vi "Network_Main.vi"(8 "error in (no error)":errorcluster, 11 "DevInfo":T1={"Hostname"="", "IPAddress"="", "MAC"="", "SerialNum"="", "Model"="", "Status"="", "FW"="", "OSDesc"="", "ImgTitle"="", "ImgDesc"="", "ImgVer"="", "ImgID"="", "IP Address Request Mode"=1, "SubnetMask"="", "Gateway"="", "DNSServer"=""} {"IP Address Request Mode" items=["Static"=1, "DHCP/Link-Local"=2, "Link-Local Only"=4, "DHCP Only"=8]}) -> (0 "error out":errorcluster, 3 "Cancelled":bool)   [LabVIEW 2021]
uses:
  TypeDefs/DevInfo.ctl
  1feb173d-b457-4ebd-b016-741c425a2058.vi
  3503507e-3d8e-4ae6-b018-2cfbcbcbc3e1.vi
  7f23f98b-f62e-4c84-a499-f9e01871bdb8.vi
  d7740b82-8dfd-4b86-b168-3c102f68faa4.vi
  36928e67-3434-4745-8582-0b47ffec617e.vi
  333e741c-c09c-4afd-acb8-9a738d66323c.vi
  7c5289c9-eb46-4be9-a5cb-af584f789a3a.vi
  ee792d3c-066e-446b-8644-9ff67b395601.vi
  <userlib>/S2 Labs/Error Reporting/ER Global.vi
  <userlib>/S2 Labs/Error Reporting/Error Reporting Class/subVIs/Report Error.vi
panel:
  in  "Cancel":bool
  in  "Apply Settings":bool
  in  "IP Mode":i32(ring) items=["Static"=1, "DHCP/Link-Local"=2, "Link-Local Only"=4, "DHCP Only"=8]
  in  "DNS.4":u8
  in  "DNS.3":u8
  in  "DNS.2":u8
  in  "DNS.1":u8 caption="DNS"
  in  "GW.4":u8
  in  "GW.3":u8
  in  "GW.2":u8
  in  "GW.1":u8 caption="Gateway"
  in  "Mask.4":u8
  in  "Mask.3":u8
  in  "Mask.2":u8
  in  "Mask.1":u8 caption="Subnet Mask"
  in  "IP.4":u8
  in  "IP.3":u8
  in  "IP.2":u8
  in  "IP.1":u8 caption="IP Address"
  in  "Hostname":string
  # "."
  # "."
  # "."
  # "."
  # "."
  # "."
  # "."
  # "."
  # "."
  # "."
  # "."
  # "."
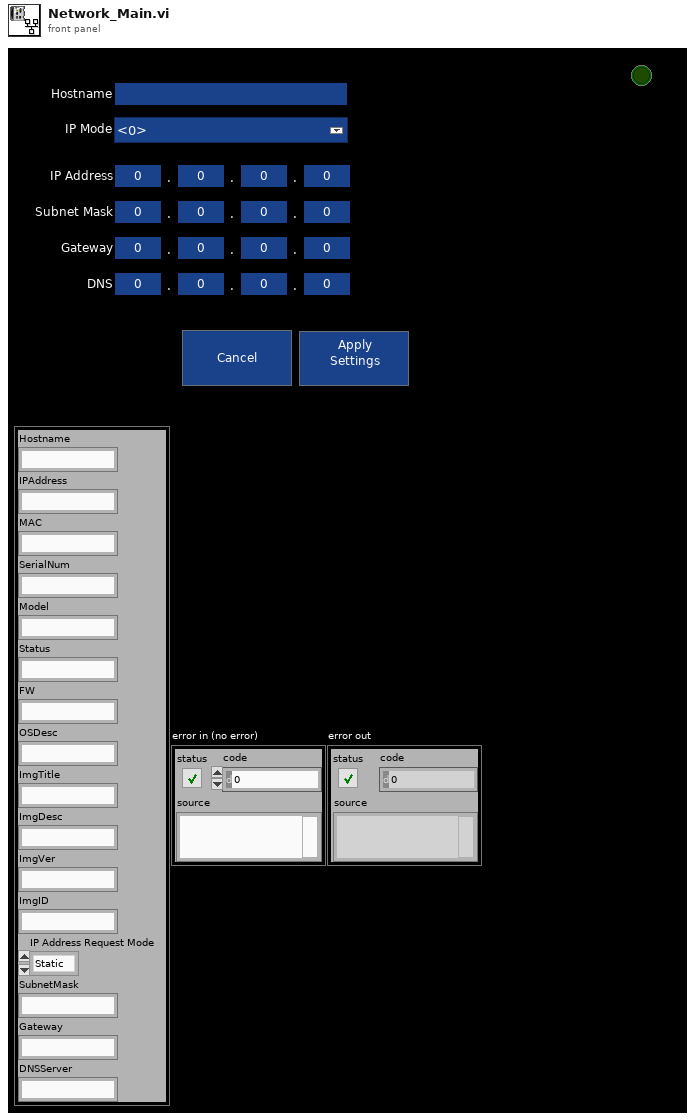
[diagram p1: front panel]
types:
  T1 = typedef "DevInfo.ctl" = cluster{"Hostname":string, "IPAddress":string, "MAC":string, "SerialNum":string, "Model":string, "Status":string, "FW":string, "OSDesc":string, "ImgTitle":string, "ImgDesc":string, "ImgVer":string, "ImgID":string, "IP Address Request Mode":i32, "SubnetMask":string, "Gateway":string, "DNSServer":string}
  T2 = enum8{"Enabled", "Disabled", "Disabled and Grayed Out"}
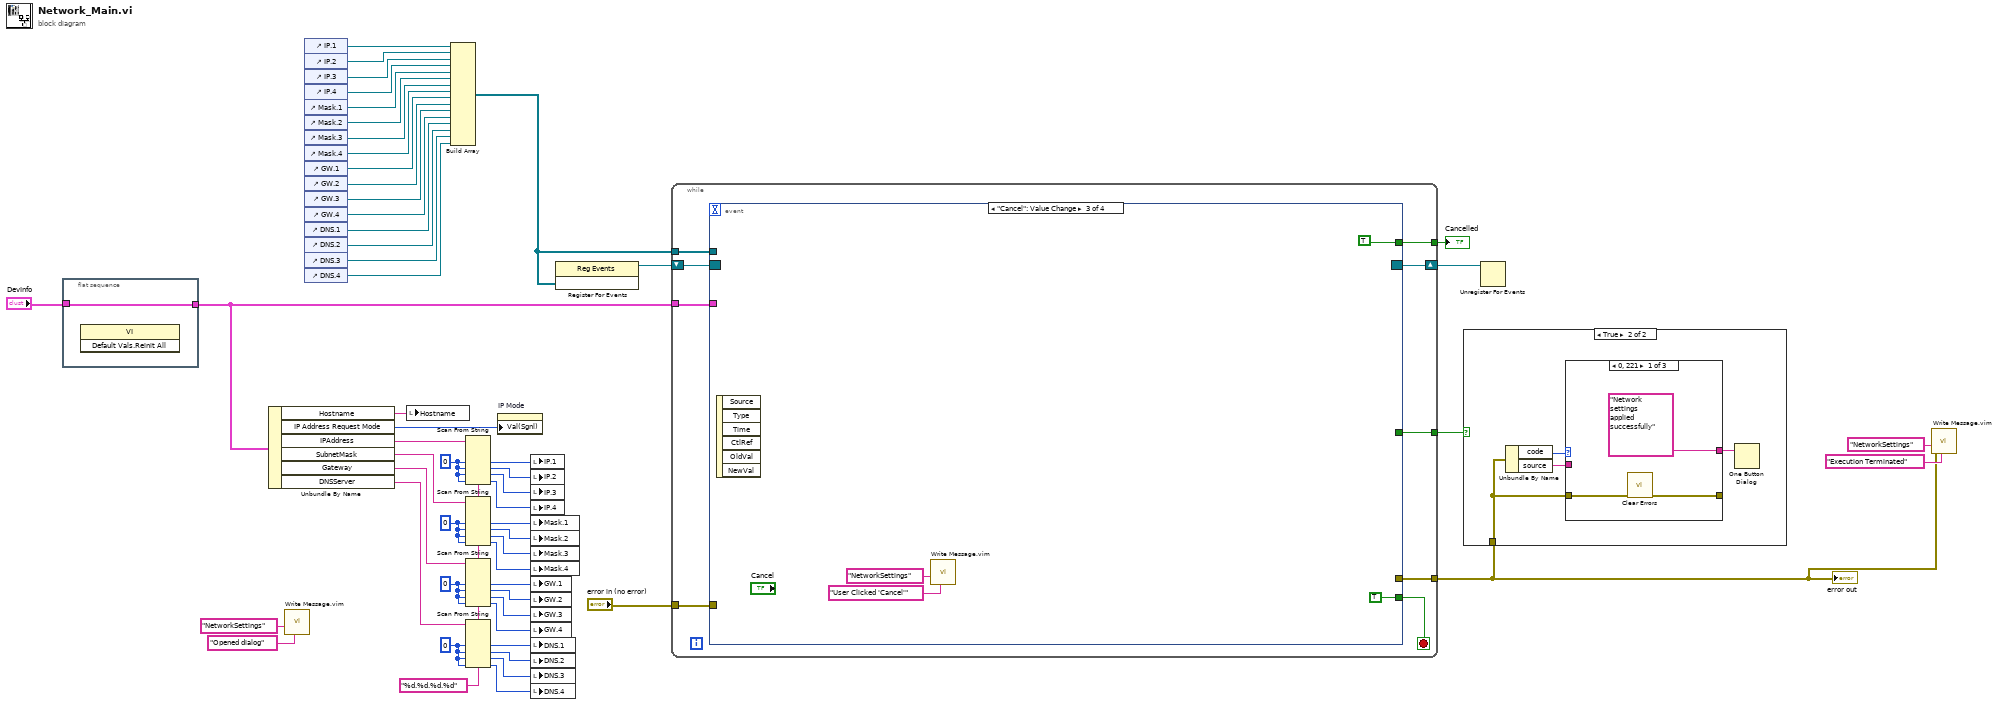
[diagram p0: block diagram]
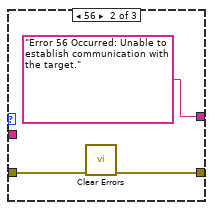
[diagram p3: hidden frame]
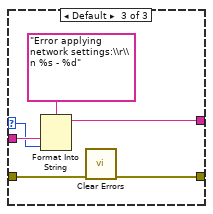
[diagram p4: hidden frame]
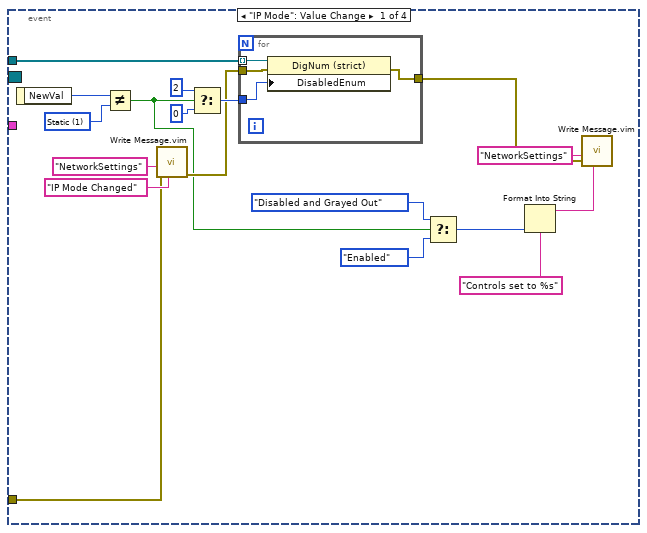
[diagram p5: hidden frame]
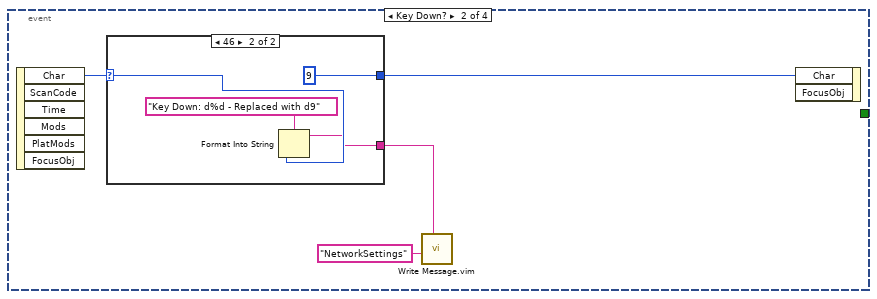
[diagram p6: hidden frame]
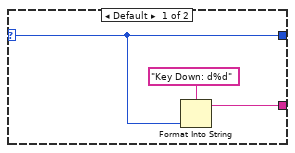
[diagram p7: hidden frame]
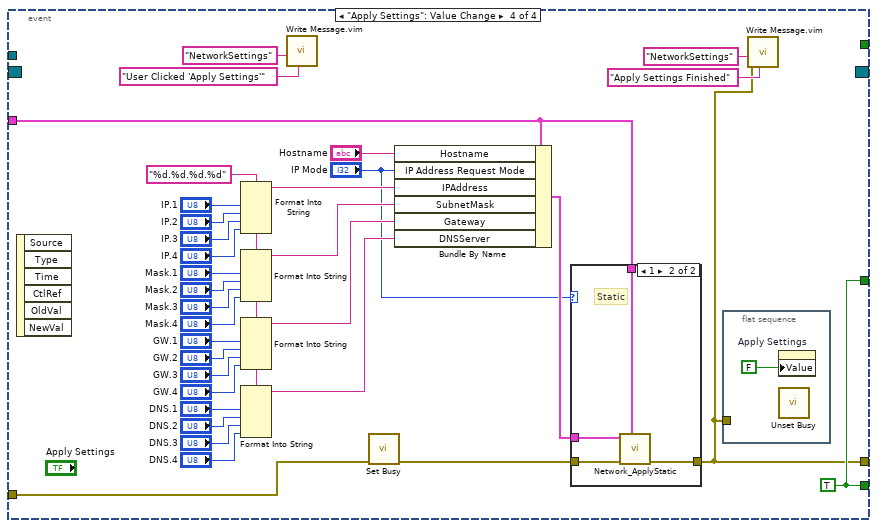
[diagram p8: hidden frame]
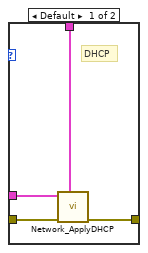
[diagram p9: hidden frame]
diagram:
  w47 = u8 0 ("default value 1")
  w48 = u8 0 ("default value 1")
  w49 = u8 0 ("default value 1")
  w55 = u8 0 ("default value 1")
  w46 = "%d.%d.%d.%d" ("format string")
  n1 = flat-sequence {
    tunnel: "DevInfo" -> [w57]
    tunnel: [w57] -> w7
    frame #0 {
      n2 = invoke class="VI" method="Default Vals.Reinit All"() -> ()  [unwired: 3 in, 3 out]
    }
  }
  n3 = Unbundle By Name(w7) -> ("Hostname"=w56:string, "IP Address Request Mode"=w30:i32, "IPAddress"=w54:string, "SubnetMask"=w33:string, "Gateway"=w32:string, "DNSServer"=w31:string)
  n4 = call "Write Message.vim"("Message Tag"="Opened dialog", "Message (string)"="NetworkSettings") -> ()  [unwired: 9 in, 1 out]
  n5 = control-ref of="IP.1"() -> (w29:refnum<vi>)
  n6 = control-ref of="IP.2"() -> (w28:refnum<vi>)
  n7 = control-ref of="IP.3"() -> (w27:refnum<vi>)
  n8 = control-ref of="IP.4"() -> (w26:refnum<vi>)
  n9 = control-ref of="Mask.1"() -> (w25:refnum<vi>)
  n10 = control-ref of="Mask.2"() -> (w24:refnum<vi>)
  n11 = control-ref of="Mask.3"() -> (w23:refnum<vi>)
  n12 = control-ref of="Mask.4"() -> (w22:refnum<vi>)
  n13 = control-ref of="GW.1"() -> (w21:refnum<vi>)
  n14 = control-ref of="GW.2"() -> (w20:refnum<vi>)
  n15 = control-ref of="GW.3"() -> (w19:refnum<vi>)
  n16 = control-ref of="GW.4"() -> (w18:refnum<vi>)
  n17 = control-ref of="DNS.1"() -> (w17:refnum<vi>)
  n18 = control-ref of="DNS.2"() -> (w16:refnum<vi>)
  n19 = control-ref of="DNS.3"() -> (w15:refnum<vi>)
  n20 = control-ref of="DNS.4"() -> (w14:refnum<vi>)
  n21 = local write "Hostname"(w56) -> ()
  n22 = Build Array(w29, w28, w27, w26, w25, w24, w23, w22, w21, w20, w19, w18, w17, w16, w15, w14) -> (w13:refnum<vi>[])
  n23 = Scan From String(format string=w46, input string=w54, default 1=w55, default 2=w55, default 3=w55, default 4=w55) -> (output 1=w53:u8, output 2=w52:u8, output 3=w51:u8, output 4=w50:u8)  [unwired: 2 in, 3 out]
  n24 = Scan From String(format string=w46, input string=w33, default 1=w49, default 2=w49, default 3=w49, default 4=w49) -> (output 1=w45:u8, output 2=w44:u8, output 3=w43:u8, output 4=w42:u8)  [unwired: 2 in, 3 out]
  n25 = Scan From String(format string=w46, input string=w32, default 1=w48, default 2=w48, default 3=w48, default 4=w48) -> (output 1=w41:u8, output 2=w40:u8, output 3=w39:u8, output 4=w38:u8)  [unwired: 2 in, 3 out]
  n26 = Scan From String(format string=w46, input string=w31, default 1=w47, default 2=w47, default 3=w47, default 4=w47) -> (output 1=w37:u8, output 2=w36:u8, output 3=w35:u8, output 4=w34:u8)  [unwired: 2 in, 3 out]
  n27 = property on="IP Mode" class="Ring (strict)"("Val(Sgnl)"=w30) -> ()  [unwired: 2 in, 2 out]
  n28 = local write "IP.1"(w53) -> ()
  n29 = local write "IP.2"(w52) -> ()
  n30 = local write "IP.3"(w51) -> ()
  n31 = local write "IP.4"(w50) -> ()
  n32 = local write "Mask.1"(w45) -> ()
  n33 = local write "Mask.2"(w44) -> ()
  n34 = local write "Mask.3"(w43) -> ()
  n35 = local write "Mask.4"(w42) -> ()
  n36 = local write "GW.1"(w41) -> ()
  n37 = local write "GW.2"(w40) -> ()
  n38 = local write "GW.3"(w39) -> ()
  n39 = local write "GW.4"(w38) -> ()
  n40 = local write "DNS.1"(w37) -> ()
  n41 = local write "DNS.2"(w36) -> ()
  n42 = local write "DNS.3"(w35) -> ()
  n43 = local write "DNS.4"(w34) -> ()
  n44 = register-events(w13) -> (reference out=w12:refnum<event-registration>)  [unwired: 2 in, 1 out]
  n45 = while {
    tunnel: w7 -> [w62]
    tunnel: w13 -> [w66]
    tunnel: "error in (no error)" -> [w63]
    tunnel: [w61] -> w2
    tunnel: [w60] -> w10
    tunnel: [w59] -> w9
    shift-right: [w58] -> w1
    shift-left: w12 -> [w65]
    stop <- w64 stop-if-true
    n46 = event shown="[2] \"Cancel\": Value Change" {
      selector: w65 -> [_ _ _ _]
      dyn-events: [_ _ _ _] -> w58
      timeout: _ -> [_ _ _ _]
      tunnel: w66 -> [w84 _ _ _]
      tunnel: [_ _ TRUE w109] -> w64
      tunnel: w63 -> [w76 _ _ w110]
      tunnel: w62 -> [_ _ _ w112]
      tunnel: [_ _ _ w104] -> w61
      tunnel: [_ _ _ w109] -> w60
      tunnel: [_ _ TRUE _] -> w59
      event "IP Mode": Value Change {
        w82 = 1 items=["Static"=1, "DHCP/Link-Local"=2, "Link-Local Only"=4, "DHCP Only"=8] ("IP Address Request Mode")
        n47 = event-data() -> ("NewVal"=w83:i32)  [unwired: 1 in]
        n48 = Not Equal?(x=w83, y=w82) -> (x != y?=w73:bool)
        n49 = call "Write Message.vim"("Message Tag"="IP Mode Changed", "error in (no error)"=w76, "Message (string)"="NetworkSettings") -> ("error out"=w75:errorcluster)  [unwired: 8 in]
        n50 = Select(t=u8 2 ("Disabled"), s=w73, f=u8 0 ("Disabled")) -> (s? t:f=w79:u8)
        n51 = for {
          tunnel: w84 -> [w88] mode=indexing
          tunnel: w79 -> [w87]
          tunnel: w75 -> [w86]
          tunnel: [w85] -> w70
          n52 = property class="DigNum (strict)"(reference=w88, error in=w86, "DisabledEnum"=w87) -> (error out=w85:errorcluster)  [unwired: 1 out]
        }
        n53 = Select(t=T2."Disabled and Grayed Out" ("Disabled"), s=w73, f=T2."Enabled" ("Disabled")) -> (s? t:f=w68:T2)
        n54 = Format Into String(format string="Controls set to %s" ("Message Tag"), w68) -> (resulting string=w67:string)  [unwired: 2 in, 1 out]
        n55 = call "Write Message.vim"("Message Tag"=w67, "error in (no error)"=w70, "Message (string)"="NetworkSettings") -> ()  [unwired: 8 in, 1 out]
      }
      event Key Down? {
        n56 = event-data() -> ("Char"=w92:i16)  [unwired: 1 in, 5 out]
        n57 = case shown="46" w92 {
          selector: w92 -> [w94 w97]
          tunnel: [w94 i16 9 ("Char")] -> w91
          tunnel: [w93 w96] -> w89
          frame Default {
            n58 = Format Into String(format string="Key Down: d%d" ("Message Tag"), w94) -> (resulting string=w93:string)  [unwired: 2 in, 1 out]
          }
          frame 46 {
            n59 = Format Into String(format string="Key Down: d%d - Replaced with d9" ("Message Tag"), w97) -> (resulting string=w96:string)  [unwired: 2 in, 1 out]
          }
        }
        n60 = call "Write Message.vim"("Message Tag"=w89, "Message (string)"="NetworkSettings") -> ()  [unwired: 9 in, 1 out]
        n61 = event-data("Char"=w91) -> ()  [unwired: 2 in, 1 out]
      }
      event "Cancel": Value Change {
        n62 = event-data() -> ()  [unwired: 1 in, 6 out]
        n63 = call "Write Message.vim"("Message Tag"="User Clicked 'Cancel'", "Message (string)"="NetworkSettings") -> ()  [unwired: 9 in, 1 out]
      }
      event "Apply Settings": Value Change {
        w109 = TRUE
        w119 = "%d.%d.%d.%d" ("format string")
        n64 = event-data() -> ()  [unwired: 1 in, 6 out]
        n65 = Format Into String(format string=w119, "IP.1", "IP.2", "IP.3", "IP.4") -> (resulting string=w118:string)  [unwired: 2 in, 1 out]
        n66 = Format Into String(format string=w119, "Mask.1", "Mask.2", "Mask.3", "Mask.4") -> (resulting string=w117:string)  [unwired: 2 in, 1 out]
        n67 = Format Into String(format string=w119, "GW.1", "GW.2", "GW.3", "GW.4") -> (resulting string=w116:string)  [unwired: 2 in, 1 out]
        n68 = Format Into String(format string=w119, "DNS.1", "DNS.2", "DNS.3", "DNS.4") -> (resulting string=w115:string)  [unwired: 2 in, 1 out]
        n69 = call "Write Message.vim"("Message Tag"="User Clicked 'Apply Settings'", "Message (string)"="NetworkSettings") -> ()  [unwired: 9 in, 1 out]
        n70 = call <vilib>:"Set Busy.vi"("error in (no error)"=w110) -> ("error out"=w111:errorcluster)  [unwired: 9 in, 1 out]
        n71 = Bundle By Name(cluster=w112, "Hostname"="Hostname", "IP Address Request Mode"="IP Mode", "IPAddress"=w118, "SubnetMask"=w117, "Gateway"=w116, "DNSServer"=w115) -> (w114:T1)
        n72 = case shown="1" "IP Mode" {
          tunnel: w114 -> [w141 w145]
          tunnel: w112 -> [w140 w144]
          tunnel: w111 -> [w139 w143]
          tunnel: [w138 w142] -> w104
          frame Default {
            # "DHCP"
            n73 = call "Network_ApplyDHCP.vi"("DevInfo Original"=w140, "error in (no error)"=w139, "DevInfo Modified"=w141) -> ("error out"=w138:errorcluster)  [unwired: 8 in]
          }
          frame 1 {
            # "Static"
            n74 = call "Network_ApplyStatic.vi"("DevInfo Original"=w144, "error in (no error)"=w143, "DevInfo Modified"=w145) -> ("error out"=w142:errorcluster)  [unwired: 8 in]
          }
        }
        n75 = flat-sequence {
          tunnel: w104 -> [_]
          frame #0 {
            n76 = property on="Apply Settings" class="Bool (strict)"("Value"=FALSE ("Apply Settings")) -> ()  [unwired: 2 in, 2 out]
            n77 = call <vilib>:"Unset Busy.vi"() -> ()  [unwired: 11 in, 1 out]
          }
        }
        n78 = call "Write Message.vim"("Message Tag"="Apply Settings Finished", "error in (no error)"=w104, "Message (string)"="NetworkSettings") -> ()  [unwired: 8 in, 1 out]
      }
    }
  }
  "error out" <- w2
  "Cancelled" <- w9
  n79 = case shown="True" w10 {
    tunnel: w2 -> [_ w146]
    frame False {
    }
    frame True {
      n80 = Unbundle By Name(w146) -> ("code"=w148:i32, "source"=w147:string)
      n81 = case shown="0, 221" w148 {
        selector: w148 -> [_ _ w158]
        tunnel: w147 -> [_ _ w161]
        tunnel: ["Network settings applied successfully" ("source") "Error 56 Occurred: Unable to establish communication with the target." ("source") w160] -> w149
        tunnel: [w150 w153 w156] -> _
        tunnel: w146 -> [w151 w154 w157]
        frame 0, 221 {
          n82 = call <vilib>:"Clear Errors.vi"("error in (no error)"=w151) -> ("error out"=w150:errorcluster)  [unwired: 5 in, 1 out]
        }
        frame 56 {
          n83 = call <vilib>:"Clear Errors.vi"("error in (no error)"=w154) -> ("error out"=w153:errorcluster)  [unwired: 5 in, 1 out]
        }
        frame Default {
          n84 = Format Into String(format string="Error applying network settings:\\r\\n %s - %d", w161, w158) -> (resulting string=w160:string)  [unwired: 2 in, 1 out]
          n85 = call <vilib>:"Clear Errors.vi"("error in (no error)"=w157) -> ("error out"=w156:errorcluster)  [unwired: 5 in, 1 out]
        }
      }
      n86 = One Button Dialog(message=w149) -> ()  [unwired: 2 out]
    }
  }
  n87 = Unregister For Events(event registration refnum=w1) -> ()  [unwired: 1 in, 1 out]
  n88 = call "Write Message.vim"("Message Tag"="Execution Terminated", "error in (no error)"=w2, "Message (string)"="NetworkSettings") -> ()  [unwired: 8 in, 1 out]
